vi "getReturnType.vi"(8 "error in (no error)":errorcluster, 11 "ICallableInfo in":refnum<class "ICallableInfo.lvclass">) -> (0 "error out":errorcluster, 2 "Return Type out":T1 items=["ctBool"=0, "ctInt"=1, "ctFloat"=2, "ctString"=3, "ctList"=4, "ctDict"=5, "ctRatio"=6, "ctProc"=7, "ctObject"=8, "ctBinaryData"=9, "ctFunc"=10, "ctComplexNumber"=11, "ctStruct"=12, "ctEnumeration"=13, "ctUndefined"=65535], 3 "ICallableInfo out":refnum<class "ICallableInfo.lvclass">)   [LabVIEW 2022 SP3, in "openDAQ.lvlib" / "IBaseObject.lvlib" / "ICallableInfo.lvlib" / "ICallableInfo.lvclass"]
uses:
  <instrlib>/openDAQ/Public/Classes/ICallableInfo/ICallableInfo.lvclass
  <instrlib>/openDAQ/Public/Classes/ICallableInfo/ICallableInfo.lvclass/ICallableInfo.ctl
  <instrlib>/openDAQ/Binaries/Windows/x86/copendaq32.dll
  <instrlib>/openDAQ/Public/TypeDef/CoreType.ctl
  <instrlib>/openDAQ/openDAQ.lvlib
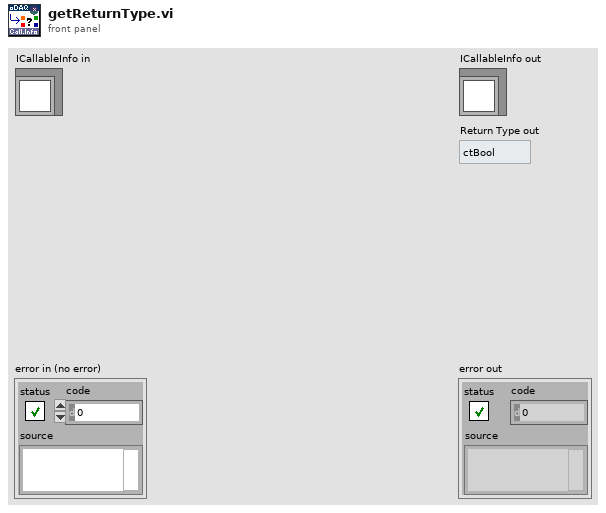
[diagram p1: front panel]
types:
  T1 = typedef "openDAQ.lvlib/CoreType.ctl" = u16
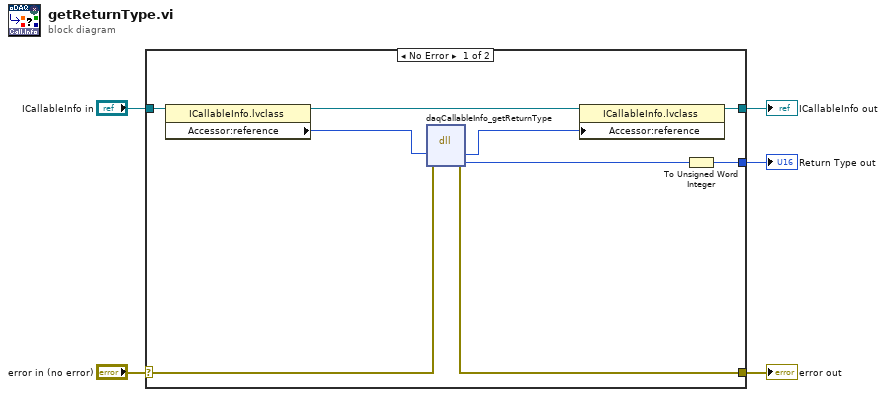
[diagram p0: block diagram]
diagram:
  n1 = case shown="No Error" "error in (no error)" {
    selector: "error in (no error)" -> [w13 w16]
    tunnel: [w12 w16] -> w4
    tunnel: [w10 w15] -> w2
    tunnel: "ICallableInfo in" -> [w14 w15]
    tunnel: [w6 _] -> w1
    frame No Error {
      n2 = property class="ICallableInfo.lvclass"(reference=w14) -> (reference out=w11:refnum<class "ICallableInfo.lvclass">, "Accessor:reference"=w9:i64)  [unwired: 1 in, 1 out]
      n3 = dll-call lib="C:/Program Files (x86)/National Instruments/LabVIEW 2022/instr.lib/openDAQ/Binaries/Windows/x86/copendaq*.*" fn="daqCallableInfo_getReturnType"(error in=w13, "callableInfo"=w9) -> (error out=w12:errorcluster, "callableInfo"=w8:i64, "type"=w7:i64)  [unwired: 4 in, 1 out]
      n4 = property class="ICallableInfo.lvclass"(reference=w11, "Accessor:reference"=w8) -> (reference out=w10:refnum<class "ICallableInfo.lvclass">)  [unwired: 1 in, 1 out]
      n5 = To Unsigned Word Integer(number=w7) -> (unsigned 16bit integer=w6:u16)
    }
    frame Error {
    }
  }
  "error out" <- w4
  "ICallableInfo out" <- w2
  "Return Type out" <- w1
